vi "FGV_login.vi"(4 "current_access_level":refnum<vi>, 6 "current_username":refnum<vi>, 7 "options":T1, 8 "error_in":errorcluster, 10 "access_level_in":i32, 11 "username_in":string) -> (0 "error_out":errorcluster, 2 "access_level_out":i32, 3 "username_out":string)   [LabVIEW 2019]
uses:
  FGV_login.ctl
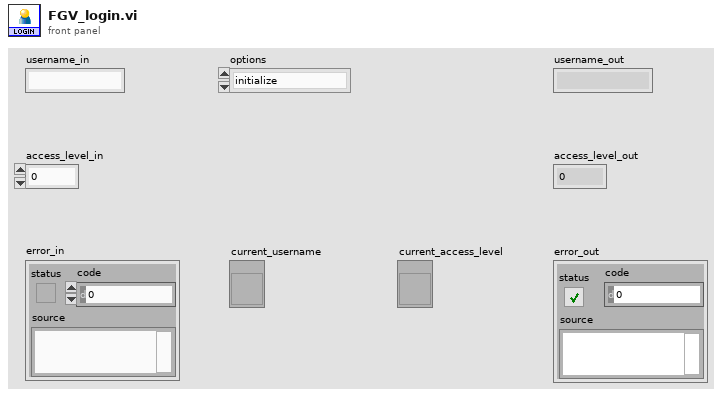
[diagram p1: front panel]
types:
  T1 = typedef "FGV_login.ctl" = enum16{"initialize", "login", "logout", "get_login_info"}
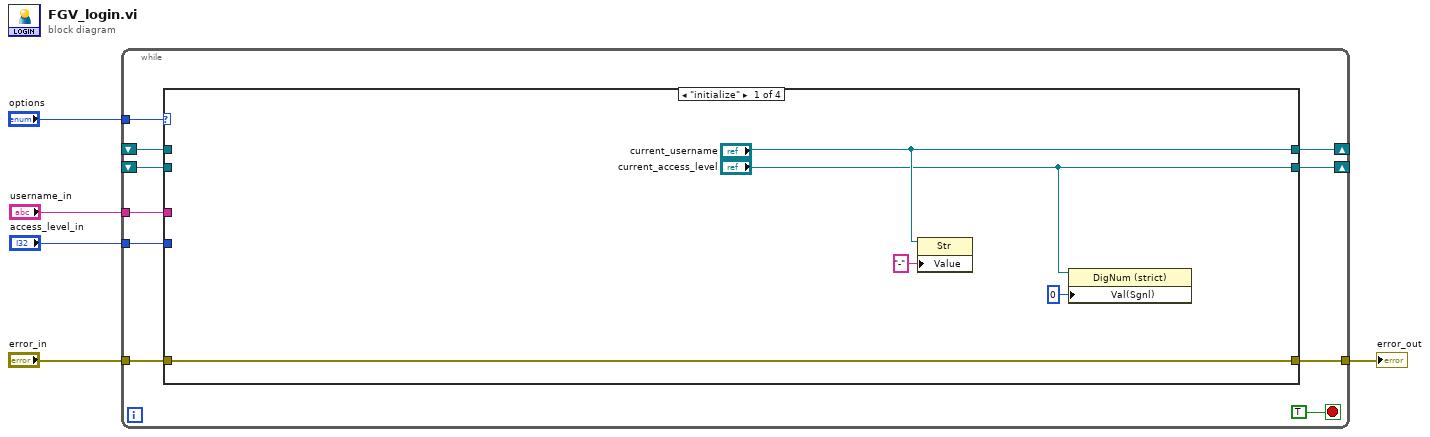
[diagram p0: block diagram]
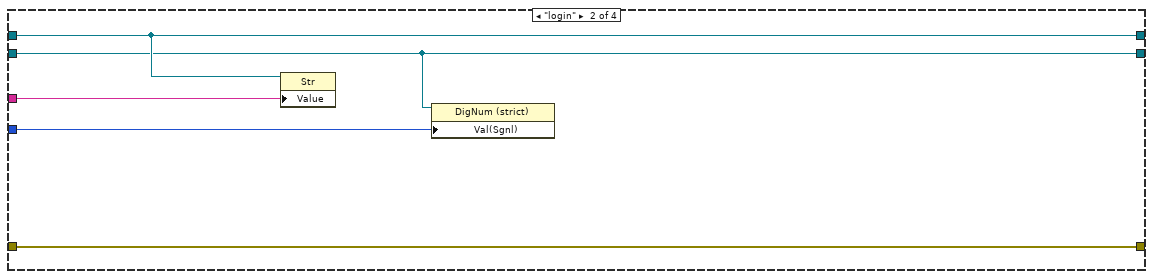
[diagram p2: hidden frame]
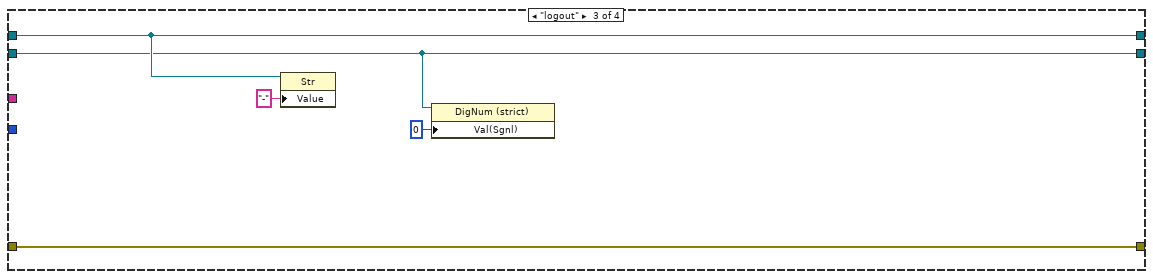
[diagram p3: hidden frame]
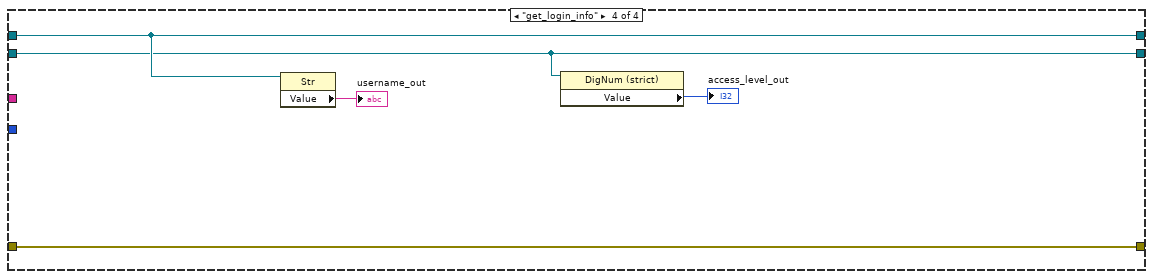
[diagram p4: hidden frame]
diagram:
  n1 = while {
    tunnel: "options" -> [w14]
    tunnel: [w13] -> w5
    tunnel: "error_in" -> [w12]
    shift-right: [w11] -> _
    shift-left: _ -> [w10]
    shift-right: [w9] -> _
    shift-left: _ -> [w8]
    tunnel: "username_in" -> [w7]
    tunnel: "access_level_in" -> [w6]
    stop <- TRUE stop-if-true
    n2 = case shown="\"initialize\"" w14 {
      tunnel: [w20 w25 w30 w35] -> w13
      tunnel: w12 -> [w20 w25 w30 w35]
      tunnel: ["current_username" w24 w29 w34] -> w11
      tunnel: w10 -> [_ w24 w29 w34]
      tunnel: ["current_access_level" w23 w28 w33] -> w9
      tunnel: w8 -> [_ w23 w28 w33]
      tunnel: w7 -> [_ w22 _ _]
      tunnel: w6 -> [_ w21 _ _]
      frame "initialize" {
        n3 = property class="Str"(reference="current_username", "Value"="-") -> ()  [unwired: 1 in, 2 out]
        n4 = property class="DigNum (strict)"(reference="current_access_level", "Val(Sgnl)"=0 ("Value")) -> ()  [unwired: 1 in, 2 out]
      }
      frame "login" {
        n5 = property class="Str"(reference=w24, "Value"=w22) -> ()  [unwired: 1 in, 2 out]
        n6 = property class="DigNum (strict)"(reference=w23, "Val(Sgnl)"=w21) -> ()  [unwired: 1 in, 2 out]
      }
      frame "logout" {
        n7 = property class="Str"(reference=w29, "Value"="-") -> ()  [unwired: 1 in, 2 out]
        n8 = property class="DigNum (strict)"(reference=w28, "Val(Sgnl)"=0 ("Value")) -> ()  [unwired: 1 in, 2 out]
      }
      frame "get_login_info" {
        n9 = property class="Str"(reference=w34) -> ("Value"=→"username_out":string)  [unwired: 1 in, 2 out]
        n10 = property class="DigNum (strict)"(reference=w33) -> ("Value"=→"access_level_out":i32)  [unwired: 1 in, 2 out]
      }
    }
  }
  "error_out" <- w5
